vi "ui_Library Error Log Window.vi"(1 "error message":string) -> ()   [LabVIEW 2012]
panel:
  out "logging console":string
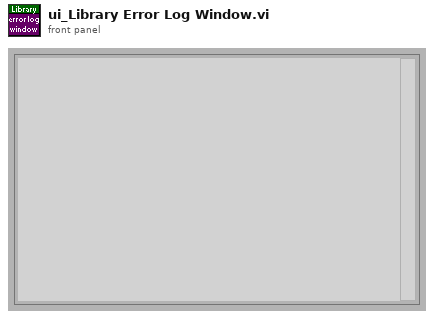
[diagram p1: front panel]
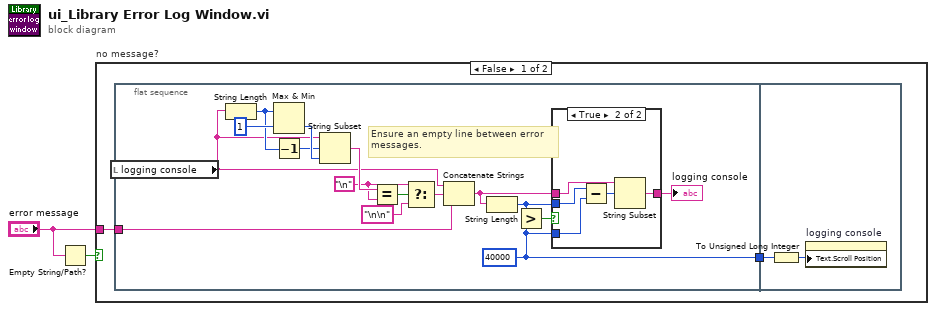
[diagram p0: block diagram]
diagram:
  n1 = Empty String/Path?(string/path="error message") -> (empty?=w2:bool)
  n2 = case "no message?" shown="False" w2 {
    tunnel: "error message" -> [w3 _]
    frame False {
      n3 = flat-sequence {
        tunnel: [w6] -> w4
        tunnel: w3 -> [w5]
        tunnel: w4 -> [w28]
        frame #0 {
          w13 = "\n"
          w6 = 40000 ("y")
          # "Ensure an empty line between error\nmessages."
          n4 = local read "logging console"() -> (w10:string)
          n5 = String Length(string=w10) -> (length=w16:i32)
          n6 = Max & Min(x=w16, y=1) -> (min(x,y)=w18:i32)  [unwired: 1 out]
          n7 = Decrement(x=w16) -> (x-1=w17:i32)
          n8 = String Subset(string=w10, offset (0)=w17, length (rest)=w18) -> (substring=w15:string)
          n9 = Equal?(x=w15, y=w13) -> (x = y?=w14:bool)
          n10 = Select(t=w13, s=w14, f="\n\n") -> (s? t:f=w11:string)
          n11 = Concatenate Strings(w10, w11, w5) -> (w9:string)
          n12 = String Length(string=w9) -> (length=w7:i32)
          n13 = Greater?(x=w7, y=w6) -> (0:w8:bool)
          n14 = case shown="True" w8 {
            tunnel: [w21 w25] -> w20
            tunnel: w9 -> [w21 w24]
            tunnel: w7 -> [_ w23]
            tunnel: w6 -> [_ w22]
            frame False {
            }
            frame True {
              n15 = Subtract(x=w23, y=w22) -> (x-y=w26:i32)
              n16 = String Subset(string=w24, offset (0)=w26) -> (substring=w25:string)  [unwired: 1 in]
            }
          }
          "logging console" <- w20
        }
        frame #1 {
          n17 = To Unsigned Long Integer(number=w28) -> (unsigned 32bit integer=w27:u32)
          n18 = property on="logging console" class="Str"("Text.Scroll Position"=w27) -> ()  [unwired: 2 in, 2 out]
        }
      }
    }
    frame True {
    }
  }
